vi "TCPGetProcessJSON.vi"(8 "error in (no error)":errorcluster, 11 "connection ID":refnum<k5>) -> ()   [LabVIEW 2013]
panel:
  out "FormattedResponse":string
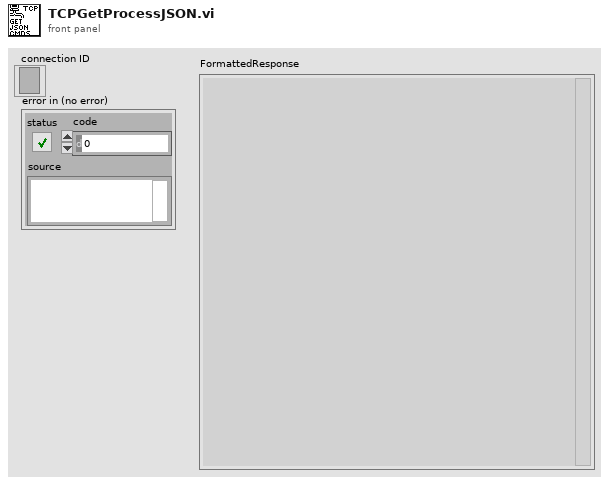
[diagram p1: front panel]
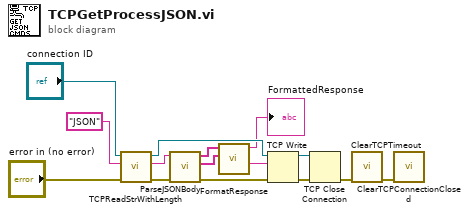
[diagram p0: block diagram]
diagram:
  n1 = call "TCPReadStrWithLength.vi"("error in (no error)"="error in (no error)", "command"="JSON", "connection ID"="connection ID") -> ("error out"=w15:errorcluster, "TCP String"=w14:string, "connection ID out"=w5:refnum<k5>)  [unwired: 6 in]
  n2 = call "ParseJSONBody.vi"("error in (no error)"=w15, "JSON object in"=w14) -> ("error out"=w10:errorcluster, "JSON Error Strings"=w12:string[], "JSON Response Strings"=w13:string[])  [unwired: 7 in]
  n3 = call "FormatResponse.vi"("JSON Error Strings"=w12, "JSON Response Strings"=w13) -> ("ResponseWithLength"=w11:string, "FormattedResponse"=→"FormattedResponse":string)  [unwired: 7 in, 1 out]
  n4 = TCP Write(connection ID=w5, data in=w11, error in (no error)=w10) -> (connection ID out=w6:refnum<k5>, error out=w7:errorcluster)  [unwired: 1 in, 1 out]
  n5 = TCP Close Connection(connection ID=w6, error in (no error)=w7) -> (error out=w8:errorcluster)  [unwired: 1 in, 1 out]
  n6 = call "ClearTCPTimeout.vi"("error in (no error)"=w8) -> ("error out"=w9:errorcluster)  [unwired: 9 in, 1 out]
  n7 = call "ClearTCPConnectionClosed.vi"("error in (no error)"=w9) -> ()  [unwired: 9 in, 2 out]
